vi "one element of zero (CDB).vi"(10 "Array in":cdb[](array[numeric])) -> (2 "equal [0]?":bool)   [LabVIEW 2020, in "NI_AALPro.lvlib"]
uses:
  NI_AALPro.lvlib
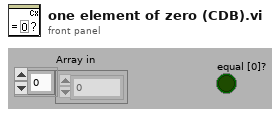
[diagram p1: front panel]
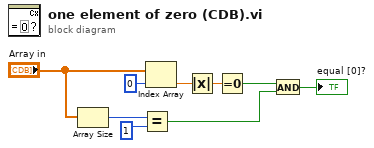
[diagram p0: block diagram]
diagram:
  n1 = Array Size(array="Array in") -> (size(s)=w8:i32)
  n2 = Equal?(x=w8, y=1) -> (x = y?=w4:bool)
  n3 = Index Array(array="Array in", index=0) -> (element=w2:cdb)
  n4 = Absolute Value(x=w2) -> (abs(x)=w1:dbl)
  n5 = Equal To 0?(x=w1) -> (x = 0?=w5:bool)
  n6 = And(x=w5, y=w4) -> (x .and. y?=→"equal [0]?":bool)
